vi "Configure Sample Clock Output Enabled [SC].vi"(8 "error in (no error)":errorcluster, 9 "Sample Clock Output Enabled (Disabled)":bool caption="sample clock output enabled (Disabled)", 11 "CS++Fgen in":refnum<class "CS++Fgen.lvclass">) -> (0 "error out":errorcluster, 3 "CS++Fgen out":refnum<class "CS++Fgen.lvclass">)   [LabVIEW 2013, in "CS++Fgen.lvlib" / "CS++Fgen.lvclass"]
doc: "This VI configures whether the sample clock appears at the sample clock output of the generator.\n\nNote:\n\n(1) This VI is part of the IviFgenSampleClock [SC] extension group."
uses:
  CS++Fgen.lvclass
  Core/Classes/CS++ProcessVariables/ProcessVariable/PV.lvclass
  Core/Classes/CS++ProcessVariables/ProcessVariable/PV.lvclass/PV.ctl
  CS++Fgen.lvclass/CS++Fgen.ctl
  Core/Classes/CS++ProcessVariables/PVConnection/PVConnection.lvclass
  Core/Classes/CS++ProcessVariables/ProcessVariable/Write Data.vi
  Core/Classes/CS++ProcessVariables/ProcessVariable/Write Timestamp.vi
  Core/Classes/CS++ProcessVariables/ProcessVariable/Write Quality.vi
  Core/Classes/CS++ProcessVariables/ProcessVariable/Write status.vi
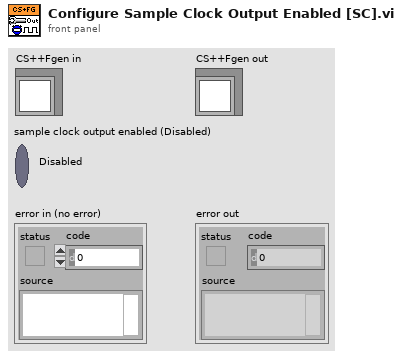
[diagram p1: front panel]
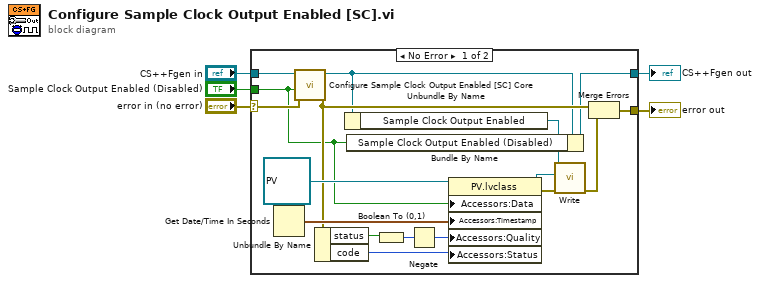
[diagram p0: block diagram]
diagram:
  n1 = case shown="No Error" "error in (no error)" {
    selector: "error in (no error)" -> [w21 w24]
    tunnel: [w6 w24] -> w4
    tunnel: [w7 w23] -> w2
    tunnel: "CS++Fgen in" -> [w22 w23]
    tunnel: "Sample Clock Output Enabled (Disabled)" -> [w10 _]
    frame No Error {
      n2 = Get Date/Time In Seconds() -> (seconds since 1Jan1904=w20:timestamp)
      n3 = call-dynamic "Configure Sample Clock Output Enabled [SC] Core.vi"("error in (no error)"=w21, "Sample Clock Output Enabled (Disabled)"=w10, "CS++Fgen in"=w22) -> ("error out"=w11:errorcluster, "CS++Fgen out"=w8:refnum<class "CS++Fgen.lvclass">)  [unwired: 7 in]
      n4 = Unbundle By Name(w11) -> ("status"=w15:bool, "code"=w13:i32)
      n5 = Unbundle By Name(w8) -> ("Sample Clock Output Enabled"=w9:refnum<class "PVConnection.lvclass">)
      n6 = Bundle By Name(cluster=w8, "Sample Clock Output Enabled (Disabled)"=w10) -> (w7:refnum<class "CS++Fgen.lvclass">)
      n7 = Boolean To (0,1)(Boolean=w15) -> (0, 1=w14:i16)
      n8 = Negate(x=w14) -> (-x=w12:i16)
      n9 = property class="PV.lvclass"(reference=refnum<class "PV.lvclass"> refnum ("PV"), "Accessors:Data"=w10, "Accessors:Timestamp"=w20, "Accessors:Quality"=w12, "Accessors:Status"=w13) -> (reference out=w17:refnum<class "PV.lvclass">, error out=w18:errorcluster)  [unwired: 1 in]
      n10 = call-dynamic "Write.vi"("error in (no error)"=w18, "PV"=w17, "PVConnection in"=w9) -> ("error out"=w16:errorcluster)  [unwired: 7 in, 1 out]
      n11 = Merge Errors(w11, w16) -> (w6:errorcluster)
    }
    frame Error {
    }
  }
  "error out" <- w4
  "CS++Fgen out" <- w2
